vi "Alarm.vi"(6 "Time Target (s)":dbl=10.0, 7 "Flag_RiseEdge_S1_prev":bool, 8 "Trigger_S2":bool, 11 "Trigger_S1":bool) -> (3 "Time has Elapsed":bool, 4 "Elapsed Time (s)":dbl, 5 "Flag_RiseEdge_S1":bool)   [LabVIEW 2020]
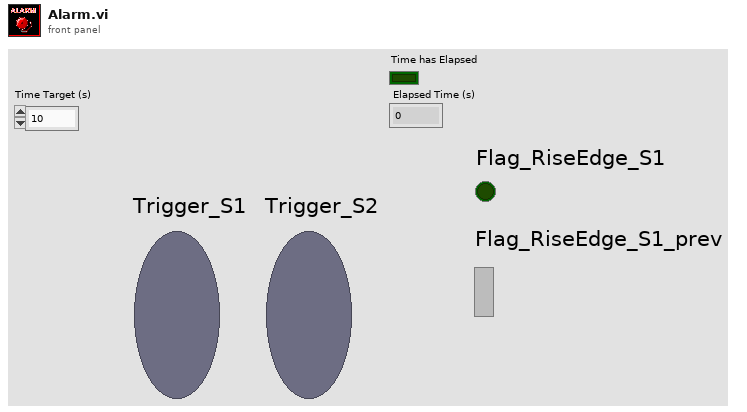
[diagram p1: front panel]
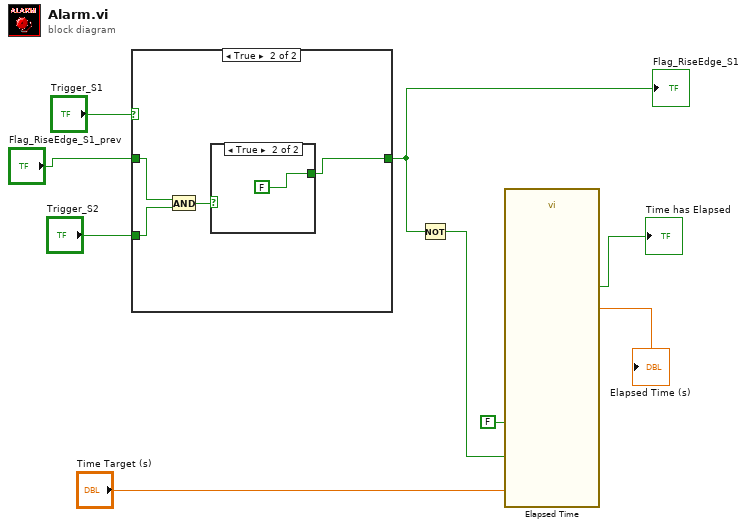
[diagram p0: block diagram]
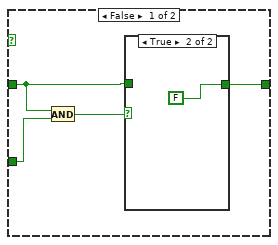
[diagram p2: hidden frame]
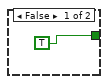
[diagram p4: hidden frame]
diagram:
  n1 = case shown="True" "Trigger_S1" {
    tunnel: [w11 w16] -> w2
    tunnel: "Flag_RiseEdge_S1_prev" -> [w10 w18]
    tunnel: "Trigger_S2" -> [w13 w17]
    frame False {
      n2 = And(x=w10, y=w13) -> (x .and. y?=w12:bool)
      n3 = case shown="True" w12 {
        tunnel: [w14 FALSE] -> w11
        tunnel: w10 -> [w14 _]
        frame False {
        }
        frame True {
        }
      }
    }
    frame True {
      n4 = And(x=w18, y=w17) -> (x .and. y?=w19:bool)
      n5 = case shown="True" w19 {
        tunnel: [TRUE FALSE] -> w16
        frame False {
        }
        frame True {
        }
      }
    }
  }
  "Flag_RiseEdge_S1" <- w2
  n6 = Not(x=w2) -> (.not. x?=w7:bool)
  n7 = call "Elapsed Time"("Time Target (s)"="Time Target (s)", "Reset"=w7, "Auto Reset"=FALSE) -> ("Elapsed Time (s)"=→"Elapsed Time (s)":dbl, "Time has Elapsed"=→"Time has Elapsed":bool)  [unwired: 9 in, 6 out]
